vi "Calculate Intersection Circles New.vi"() -> ()   [LabVIEW 2014]
panel:
  out "k":dbl
  out "p":dbl
  out "f":dbl
  out "e":dbl
  out "y2":dbl
  out "x2":dbl
  out "y1":dbl
  out "x1":dbl
  in  "r2":dbl
  in  "d":dbl
  in  "c":dbl
  in  "r1":dbl
  in  "b":dbl
  in  "a":dbl
  # "Usage:\n(a, b) signifies the (x, y) coordinates of circle 1 with radius r1.\n(c, d) signifies the (x, y) coordinates of circle 2 with radius r2.\n\nThe VI will return 4 values:\n- (x, y) coordinates where / if the circles intersect, as x1 and y1.\n- (x, y) coordinates where / if the circles intersect secondly, as x2 and y2.\n\nImportant: if the circles do not intersect 'NaN' will be returned"
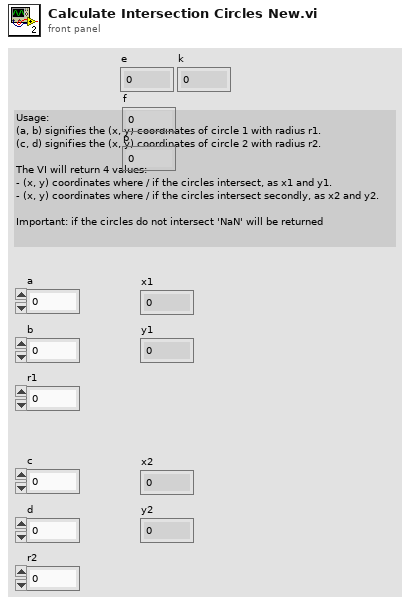
[diagram p1: front panel]
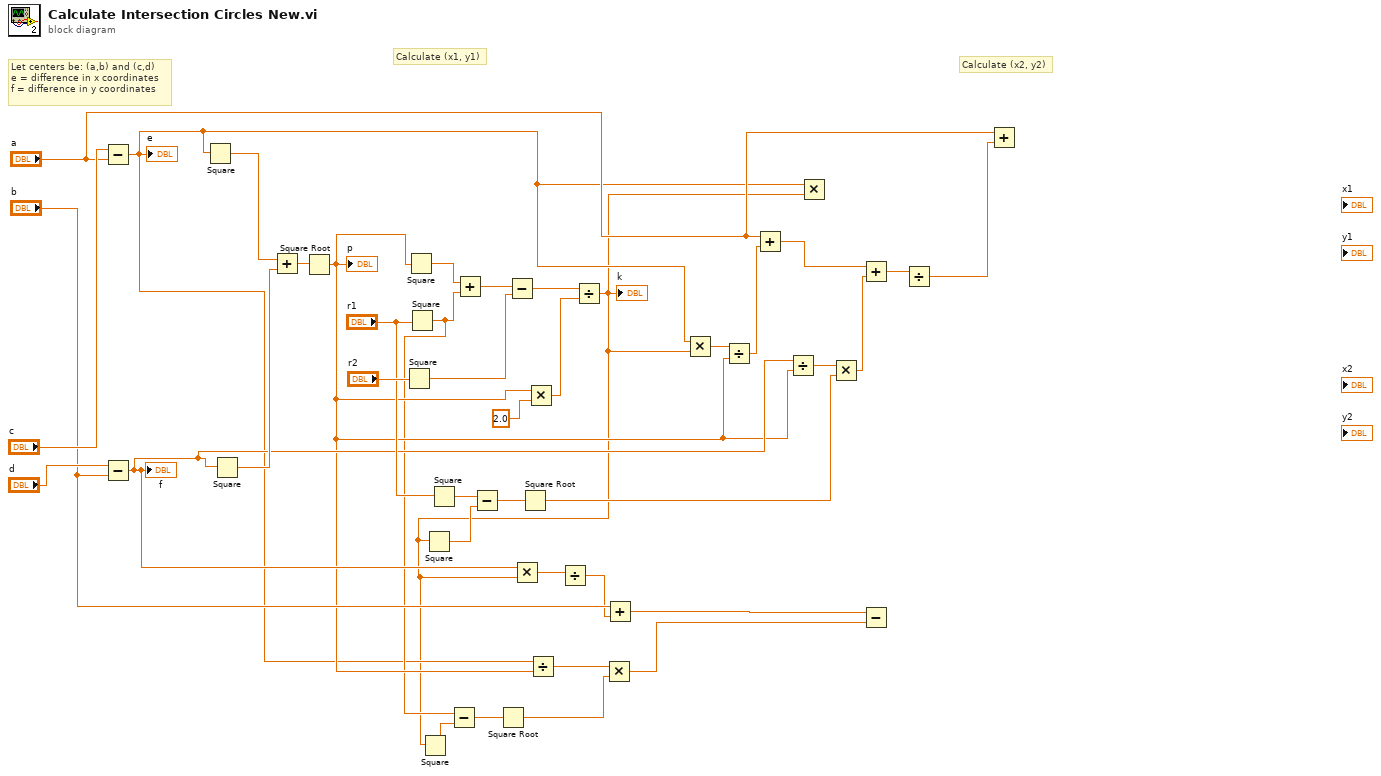
[diagram p0: block diagram]
diagram:
  # "Calculate (x2, y2)"
  # "Calculate (x1, y1)"
  # "Let centers be: (a,b) and (c,d)\ne = difference in x coordinates\nf = difference in y coordinates"
  n1 = Subtract(x="c", y="a") -> (x-y=w4:dbl)
  "e" <- w4
  n2 = Subtract(x="d", y="b") -> (x-y=w16:dbl)
  "f" <- w16
  n3 = Square(x=w4) -> (x^2=w37:dbl)
  n4 = Square(x=w16) -> (x^2=w36:dbl)
  n5 = Add(x=w37, y=w36) -> (x+y=w35:dbl)
  n6 = Square Root(x=w35) -> (sqrt(x)=w10:dbl)
  "p" <- w10
  n7 = Square(x="r2") -> (x^2=w31:dbl)
  n8 = Square(x=w10) -> (x^2=w34:dbl)
  n9 = Square(x="r1") -> (x^2=w9:dbl)
  n10 = Square(x="r1") -> (x^2=w22:dbl)
  n11 = Add(x=w34, y=w9) -> (x+y=w33:dbl)
  n12 = Subtract(x=w33, y=w31) -> (x-y=w30:dbl)
  n13 = Multiply(x=w10, y=2.0) -> (x*y=w28:dbl)
  n14 = Divide(x=w4, y=w10) -> (x/y=w11:dbl)
  n15 = Divide(x=w30, y=w28) -> (x/y=w3:dbl)
  "k" <- w3
  n16 = Square(x=w3) -> (x^2=w8:dbl)
  n17 = Square(x=w3) -> (x^2=w21:dbl)
  n18 = Subtract(x=w9, y=w8) -> (x-y=w7:dbl)
  n19 = Subtract(x=w22, y=w21) -> (x-y=w20:dbl)
  n20 = Square Root(x=w7) -> (sqrt(x)=w6:dbl)
  n21 = Multiply(x=w16, y=w3) -> (x*y=w15:dbl)
  n22 = Square Root(x=w20) -> (sqrt(x)=w19:dbl)
  n23 = Divide(x=w15) -> (x/y=w14:dbl)  [unwired: 1 in]
  n24 = Multiply(x=w11, y=w6) -> (x*y=w12:dbl)
  n25 = Add(x="b", y=w14) -> (x+y=w13:dbl)
  n26 = Multiply(x=w4, y=w3) -> (x*y=w27:dbl)
  n27 = Divide(x=w27, y=w10) -> (x/y=w26:dbl)
  n28 = Add(x="a", y=w26) -> (x+y=w25:dbl)
  n29 = Divide(x=w16, y=w10) -> (x/y=w24:dbl)
  n30 = Multiply(x=w4, y=w3) -> ()  [unwired: 1 out]
  n31 = Multiply(x=w24, y=w19) -> (x*y=w18:dbl)
  n32 = Add(x=w25, y=w18) -> (x+y=w2:dbl)
  n33 = Subtract(x=w13, y=w12) -> ()  [unwired: 1 out]
  n34 = Divide(x=w2) -> (x/y=w1:dbl)  [unwired: 1 in]
  n35 = Add(x="a", y=w1) -> ()  [unwired: 1 out]
